vi "Create-Reset counter.vi"(8 "error in (no error)":errorcluster, 11 "Counter name (dflt=blank)":string) -> (0 "error out":errorcluster)   [LabVIEW 2021, in "Named Counters.lvlib"]
uses:
  Named Counters.lvlib
  Counter Cluster.ctl
  Counter global variable.vi
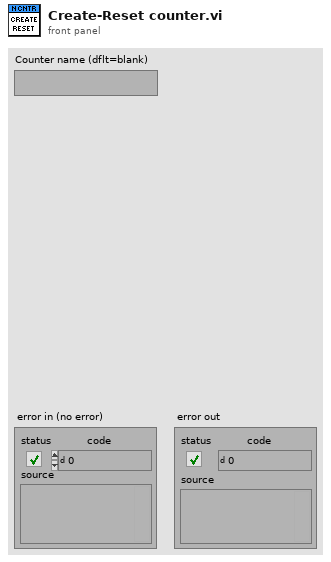
[diagram p1: front panel]
types:
  T1 = typedef "Named Counters.lvlib/Counter Cluster.ctl" = cluster{"Name":string, "Value":i32}
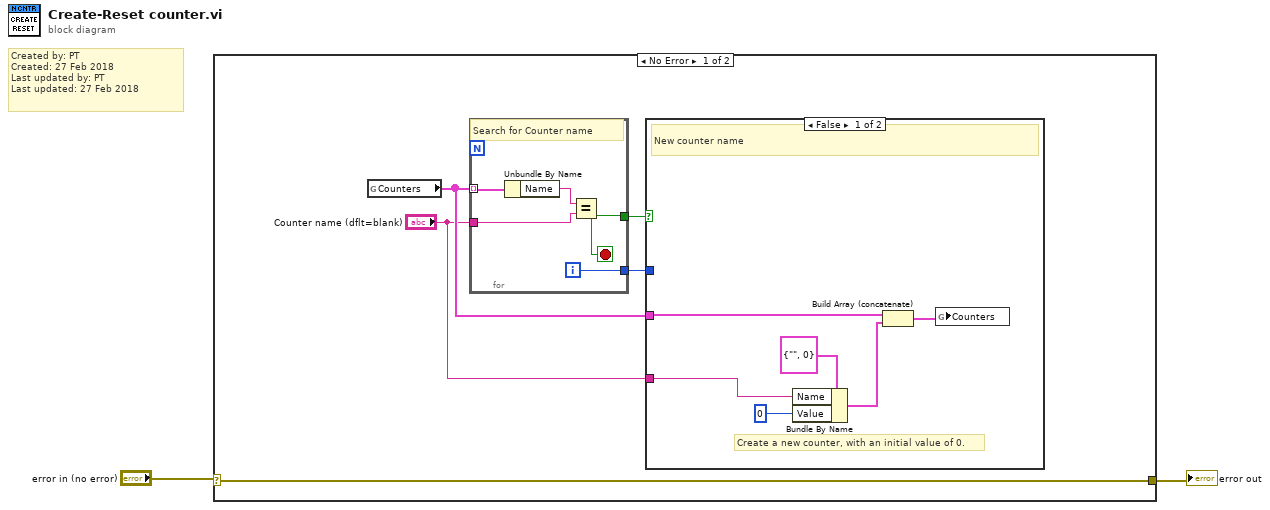
[diagram p0: block diagram]
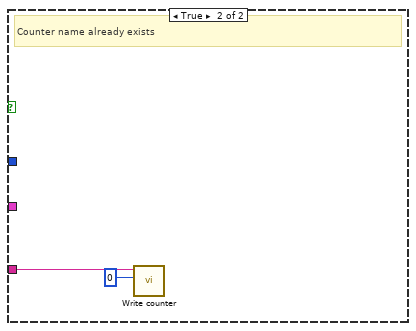
[diagram p2: hidden frame]
diagram:
  # "Created by: PT\nCreated: 27 Feb 2018\nLast updated by: PT\nLast updated: 27 Feb 2018"
  n1 = case shown="No Error" "error in (no error)" {
    selector: "error in (no error)" -> [w3 w21]
    tunnel: [w3 w21] -> w1
    frame No Error {
      n2 = global read "Counter global variable.vi" "Counters"() -> (w6:T1[])
      n3 = for {
        tunnel: w6 -> [w20] mode=indexing
        tunnel: "Counter name (dflt=blank)" -> [w18]
        tunnel: [w17] -> w7
        tunnel: [w16] -> w4
        i -> [w16]
        stop <- w17 stop-if-true
        # "Search for Counter name"
        n4 = Unbundle By Name(w20) -> ("Name"=w19:string)
        n5 = Equal?(x=w19, y=w18) -> (x = y?=w17:bool)
      }
      n6 = case shown="False" w7 {
        tunnel: w6 -> [w13 _]
        tunnel: "Counter name (dflt=blank)" -> [w11 w15]
        tunnel: w4 -> [_ _]
        frame False {
          # "Create a new counter, with an initial value of 0."
          # "New counter name"
          n7 = Bundle By Name(cluster=T1 {"Name"="", "Value"=0} ("Timer Cluster"), "Name"=w11, "Value"=0) -> (w10:T1)
          n8 = Build Array (concatenate)(w13, w10) -> (w8:T1[])
          n9 = global write "Counter global variable.vi" "Counters"(w8) -> ()
        }
        frame True {
          # "Counter name already exists"
          n10 = call "Write counter.vi"("Value"=0, "Counter name (dflt=blank)"=w15) -> ()  [unwired: 9 in, 1 out]
        }
      }
    }
    frame Error {
    }
  }
  "error out" <- w1
